vi "Galil_QR_full.vi"() -> ()   [LabVIEW 2011]
uses:
  <vilib>/Platform/TimedLoop/XDataNode/timing_clust.ctl
  <vilib>/Platform/TimedLoop/XDataNode/nitl_modes.ctl
  <vilib>/Platform/TimedLoop/XDataNode/wakeup.ctl
  <vilib>/Platform/TimedLoop/XDataNode/XDataNode.xnode
  <vilib>/Platform/TimedLoop/XDataNode/XDNodeRunTimeDep.lvlib
panel:
  in  "Galil.IGalil":refnum<k7>
  out "TIME":dbl
  out "Library Version:":string
  in  "Stop Program":bool
  out "error out":errorcluster
  out "Description":string[](array[string])
  out "Units":string[](array[string])
  out "sourceValue":dbl[](array[numeric])
  out "Number of Elements\nin Data Record":i32
  out "sources":string[](array[string])
  out "For error out":errorcluster
  out "Connected To:":string
  in  "Connection String:":string
  # "This vi shows how to access data record information using the QR method with the Galil Communications Library.  \n\nIf Connection String is left blank, the vi will open the connections dialog when run.  If a value is input into Connection String, the vi will attempt to connect to the controller at that address (ie COM1 19200).\n\nThis vi gets the full data record and constantatly updates the sourceValue, sourceUnits and sourceDescription arrays until the stop button is pressed.  This vi uses the QR method for obtaining the data record information."
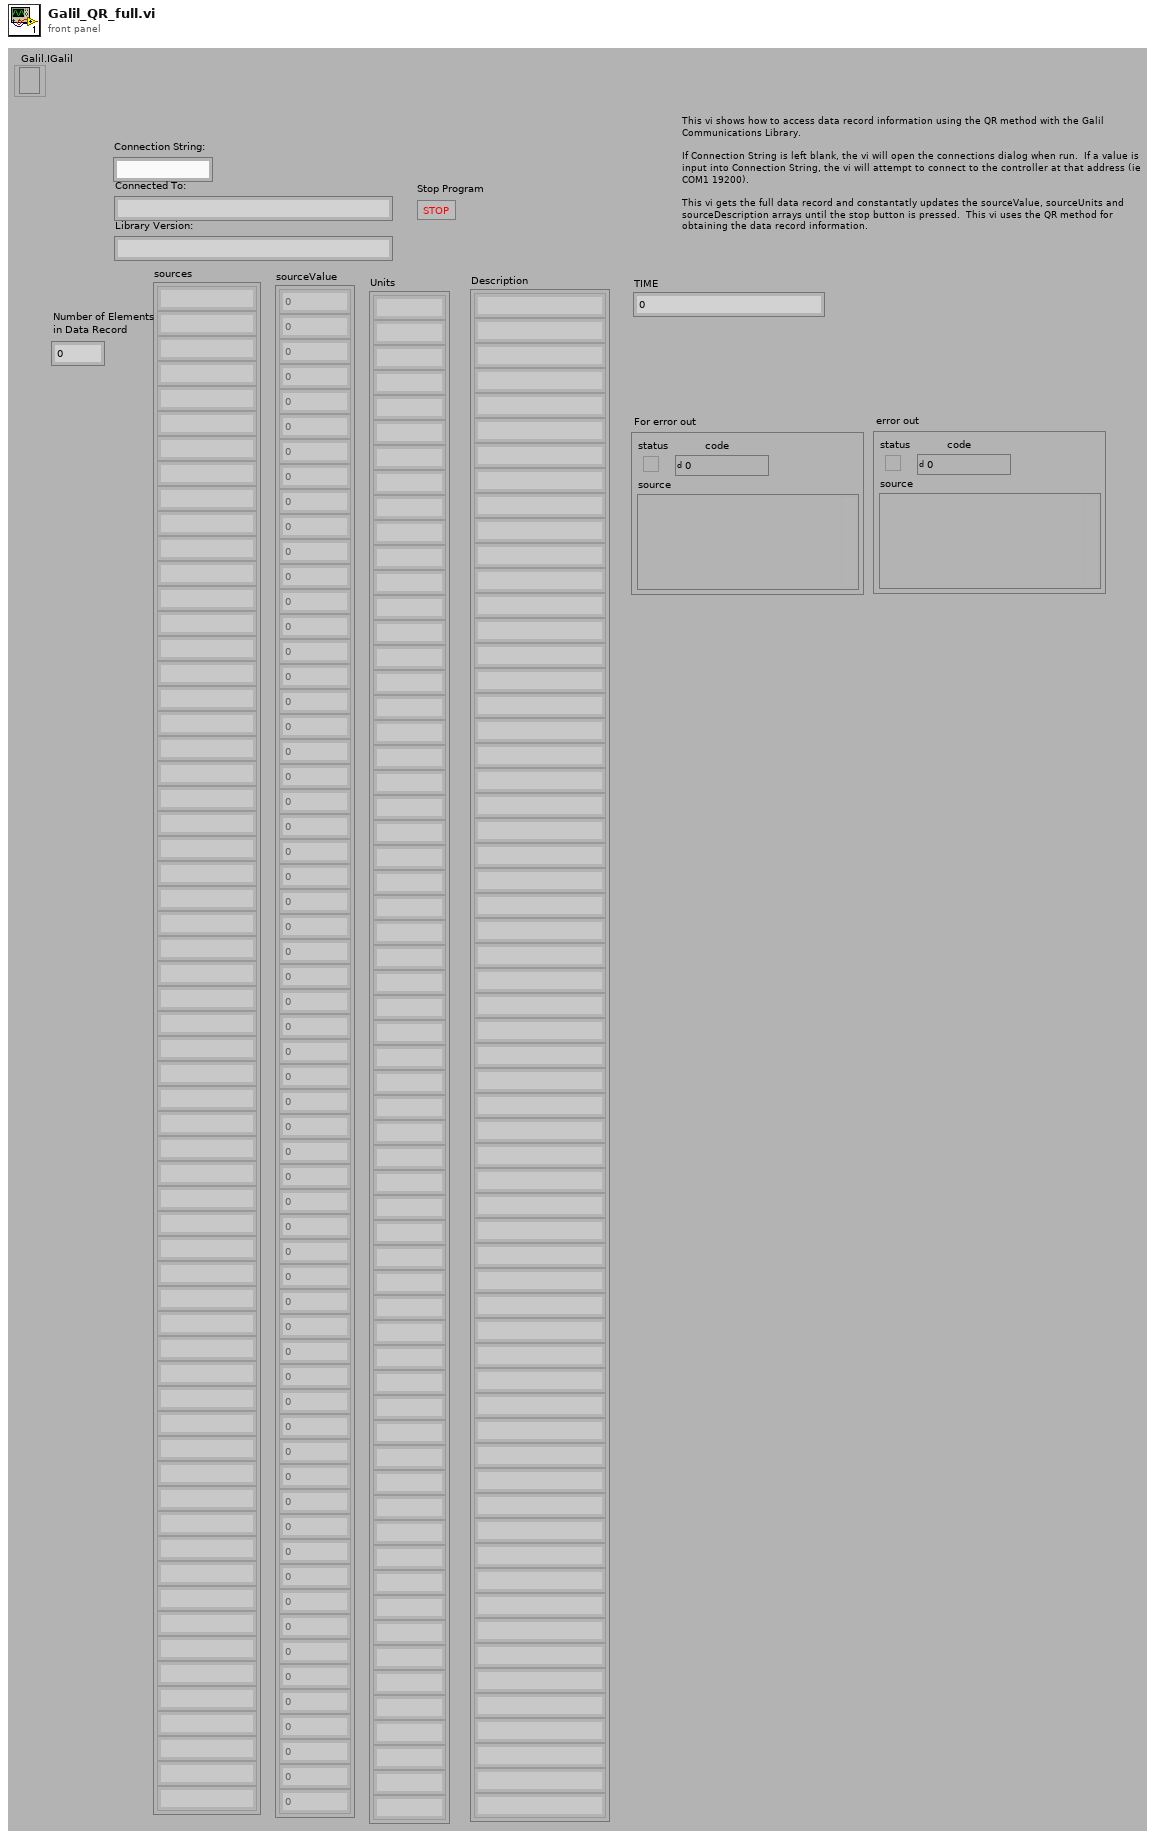
[diagram p1: front panel]
types:
  T1 = typedef "XDNodeRunTimeDep.lvlib/timing_clust.ctl" = cluster{"Expected End [f-1]":u64, "Actual End [f-1]":u64, "Finished Late? [f-1]":bool, "Expected End [i-1]":u64, "Actual End [i-1]":u64, "Finished Late? [i-1]":bool, "Expected Start [i]":u64, "Actual Start [i]":u64, "Expected Start [f]":u64, "Actual Start [f]":u64, "Source Name":string, "Structure Name":string, "Period":i64, "Deadline":i64, "Offset":i64, "Start":i64, "Priority":i32, "Timeout":i32, "Mode":T2, "Wakeup Reason":T3, "Error":errorcluster, "Source Type":string, "Secondary Source Type":string, "Global End Time":u64, "Global Start Time":u64, "Frame Duration":u64, "Iteration Duration":u64, "Assigned CPU":i32, "I/O Scan Engine Mode":u32}
  T2 = typedef "XDNodeRunTimeDep.lvlib/nitl_modes.ctl" = enum32{"No Change", "Process missed periods, maintain original phase", "Discard missed periods, maintain original phase", "Process missed periods, ignore original phase", "Discard missed periods, ignore original phase"}
  T3 = typedef "XDNodeRunTimeDep.lvlib/wakeup.ctl" = enum32{"Normal", "Aborted", "Asynchronous wakeup", "Timing source error", "Timed loop error", "Timeout"}
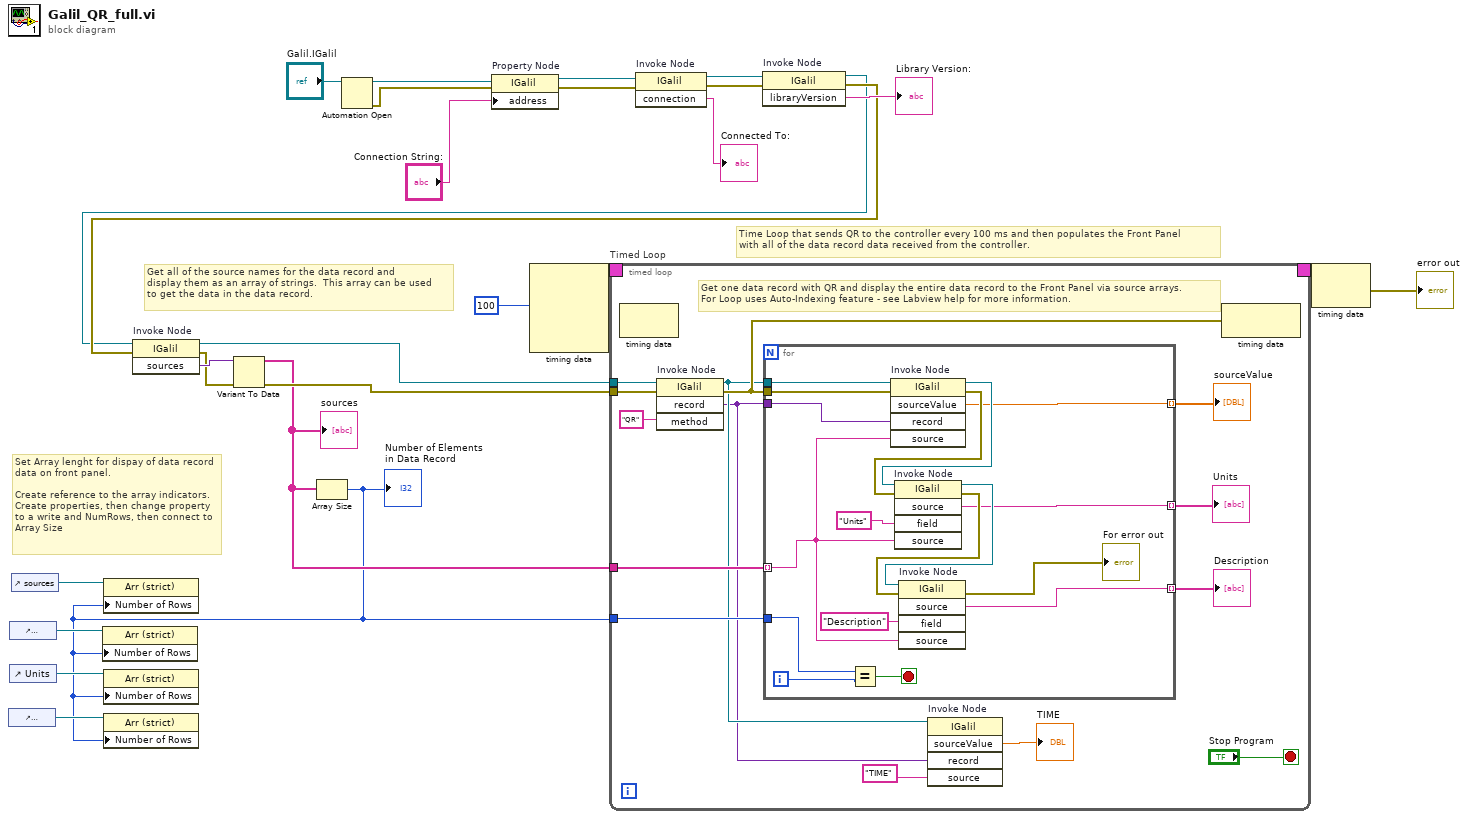
[diagram p0: block diagram]
diagram:
  # "Set Array lenght for dispay of data record \ndata on front panel.\n\nCreate reference to the array indicators.  Create properties, then change property to a write and NumRows, then connect to Array Size"
  # "Time Loop that sends QR to the controller every 100 ms and then populates the Front Panel\nwith all of the data record data received from the controller."
  # "Get all of the source names for the data record and \ndisplay them as an array of strings.  This array can be used\nto get the data in the data record."
  n1 = control-ref of="Description"() -> (w8:refnum<vi>)
  n2 = control-ref of="sourceValue"() -> (w10:refnum<vi>)
  n3 = control-ref of="Units"() -> (w9:refnum<vi>)
  n4 = control-ref of="sources"() -> (w11:refnum<vi>)
  n5 = Automation Open(Automation Refnum="Galil.IGalil") -> (Automation Refnum=w26:refnum<k7>, error out=w24:errorcluster)  [unwired: 1 in, 2 out]
  n6 = property on="Property Node" class="IGalil"(reference=w26, error in=w24, "address"="Connection String:") -> (reference out=w25:refnum<k7>, error out=w23:errorcluster)
  n7 = node-c288(100) -> (w15:T1)  [unwired: 3 out]
  n8 = invoke on="Invoke Node" class="IGalil" method="connection"(reference=w25, error in=w23) -> (reference out=w5:refnum<k7>, error out=w4:errorcluster, "connection"=→"Connected To:":string)  [unwired: 1 in]
  n9 = invoke on="Invoke Node" class="IGalil" method="libraryVersion"(reference=w5, error in=w4) -> (reference out=w2:refnum<k7>, error out=w3:errorcluster, "libraryVersion"=→"Library Version:":string)  [unwired: 1 in]
  n10 = invoke on="Invoke Node" class="IGalil" method="sources"(reference=w2, error in=w3) -> (reference out=w18:refnum<k7>, error out=w19:errorcluster, "sources"=w20:variant)  [unwired: 1 in]
  n11 = Variant To Data(error in=w19, Variant=w20) -> (data=w16:string[], error out=w17:errorcluster)  [unwired: 1 in]
  "sources" <- w16
  n12 = Array Size(array=w16) -> (size(s)=w7:i32)
  "Number of Elements\nin Data Record" <- w7
  n13 = property class="Arr (strict)"(reference=w10, "Number of Rows"=w7) -> ()  [unwired: 1 in, 2 out]
  n14 = property class="Arr (strict)"(reference=w11, "Number of Rows"=w7) -> ()  [unwired: 1 in, 2 out]
  n15 = property class="Arr (strict)"(reference=w9, "Number of Rows"=w7) -> ()  [unwired: 1 in, 2 out]
  n16 = property class="Arr (strict)"(reference=w8, "Number of Rows"=w7) -> ()  [unwired: 1 in, 2 out]
  n17 = timed-loop "Timed Loop" {
    timing: w15 -> [_]
    timing-out: [_] -> w14
    tunnel: w18 -> [w32]
    tunnel: w17 -> [w39]
    tunnel: w16 -> [w38]
    tunnel: w7 -> [w37]
    stop <- "Stop Program" stop-if-true
    # "Get one data record with QR and display the entire data record to the Front Panel via source arrays.\nFor Loop uses Auto-Indexing feature - see Labview help for more information."
    n18 = node-c288() -> ()  [unwired: 2 out]
    n19 = invoke on="Invoke Node" class="IGalil" method="record"(reference=w32, error in=w39, "method"="QR") -> (reference out=w31:refnum<k7>, error out=w33:errorcluster, "record"=w30:variant)  [unwired: 1 in, 1 out]
    n20 = for {
      tunnel: w31 -> [w57]
      tunnel: w33 -> [w56]
      tunnel: w30 -> [w51]
      tunnel: w38 -> [w42] mode=indexing
      tunnel: w37 -> [w49]
      tunnel: [w48] -> w36 mode=indexing
      tunnel: [w45] -> w35 mode=indexing
      tunnel: [w44] -> w34 mode=indexing
      i -> [w47]
      stop <- w50 stop-if-true
      n21 = Equal?(x=w49, y=w47) -> (x = y?=w50:bool)
      n22 = invoke on="Invoke Node" class="IGalil" method="sourceValue"(reference=w57, error in=w56, "record"=w51, "source"=w42) -> (reference out=w55:refnum<k7>, error out=w54:errorcluster, "sourceValue"=w48:dbl)  [unwired: 1 in, 2 out]
      n23 = invoke on="Invoke Node" class="IGalil" method="source"(reference=w55, error in=w54, "field"="Units", "source"=w42) -> (reference out=w53:refnum<k7>, error out=w52:errorcluster, "source"=w45:string)  [unwired: 1 in, 2 out]
      n24 = invoke on="Invoke Node" class="IGalil" method="source"(reference=w53, error in=w52, "field"="Description", "source"=w42) -> (error out=→"For error out":errorcluster, "source"=w44:string)  [unwired: 1 in, 3 out]
    }
    "sourceValue" <- w36
    "Units" <- w35
    "Description" <- w34
    n25 = invoke on="Invoke Node" class="IGalil" method="sourceValue"(reference=w31, "record"=w30, "source"="TIME") -> ("sourceValue"=→"TIME":dbl)  [unwired: 2 in, 4 out]
    n26 = node-c288(w33) -> ()  [unwired: 1 out]
  }
  n27 = node-c288(w14) -> (→"error out":errorcluster)
